vi "Alter Display.vi"(7 "obsticle location":dbl[](array[numeric]), 8 "error in (no error)":errorcluster, 9 "Display Map":dbl[][](array[numeric]), 10 "robot direction":string, 11 "robot location":dbl[](array[numeric])) -> (0 "error out":errorcluster, 2 "Map":u16[][](array[ring]), 3 "target location":dbl[](array[numeric]))   [LabVIEW 2015]
uses:
  <vilib>/robotics/Navigation/shared/WorldMap/OccupancyGridWorldMap/NI_Robotics_OccupancyGridWorldMap.lvclass
  <vilib>/robotics/Navigation/NI_Robotics_Navigation .lvlib
panel:
  out "Indices":i32[][](array[numeric])
  out "distances":dbl[](array[numeric])
  out "Priority level array":dbl[][](array[numeric])
  out "route map":dbl[][](array[numeric])
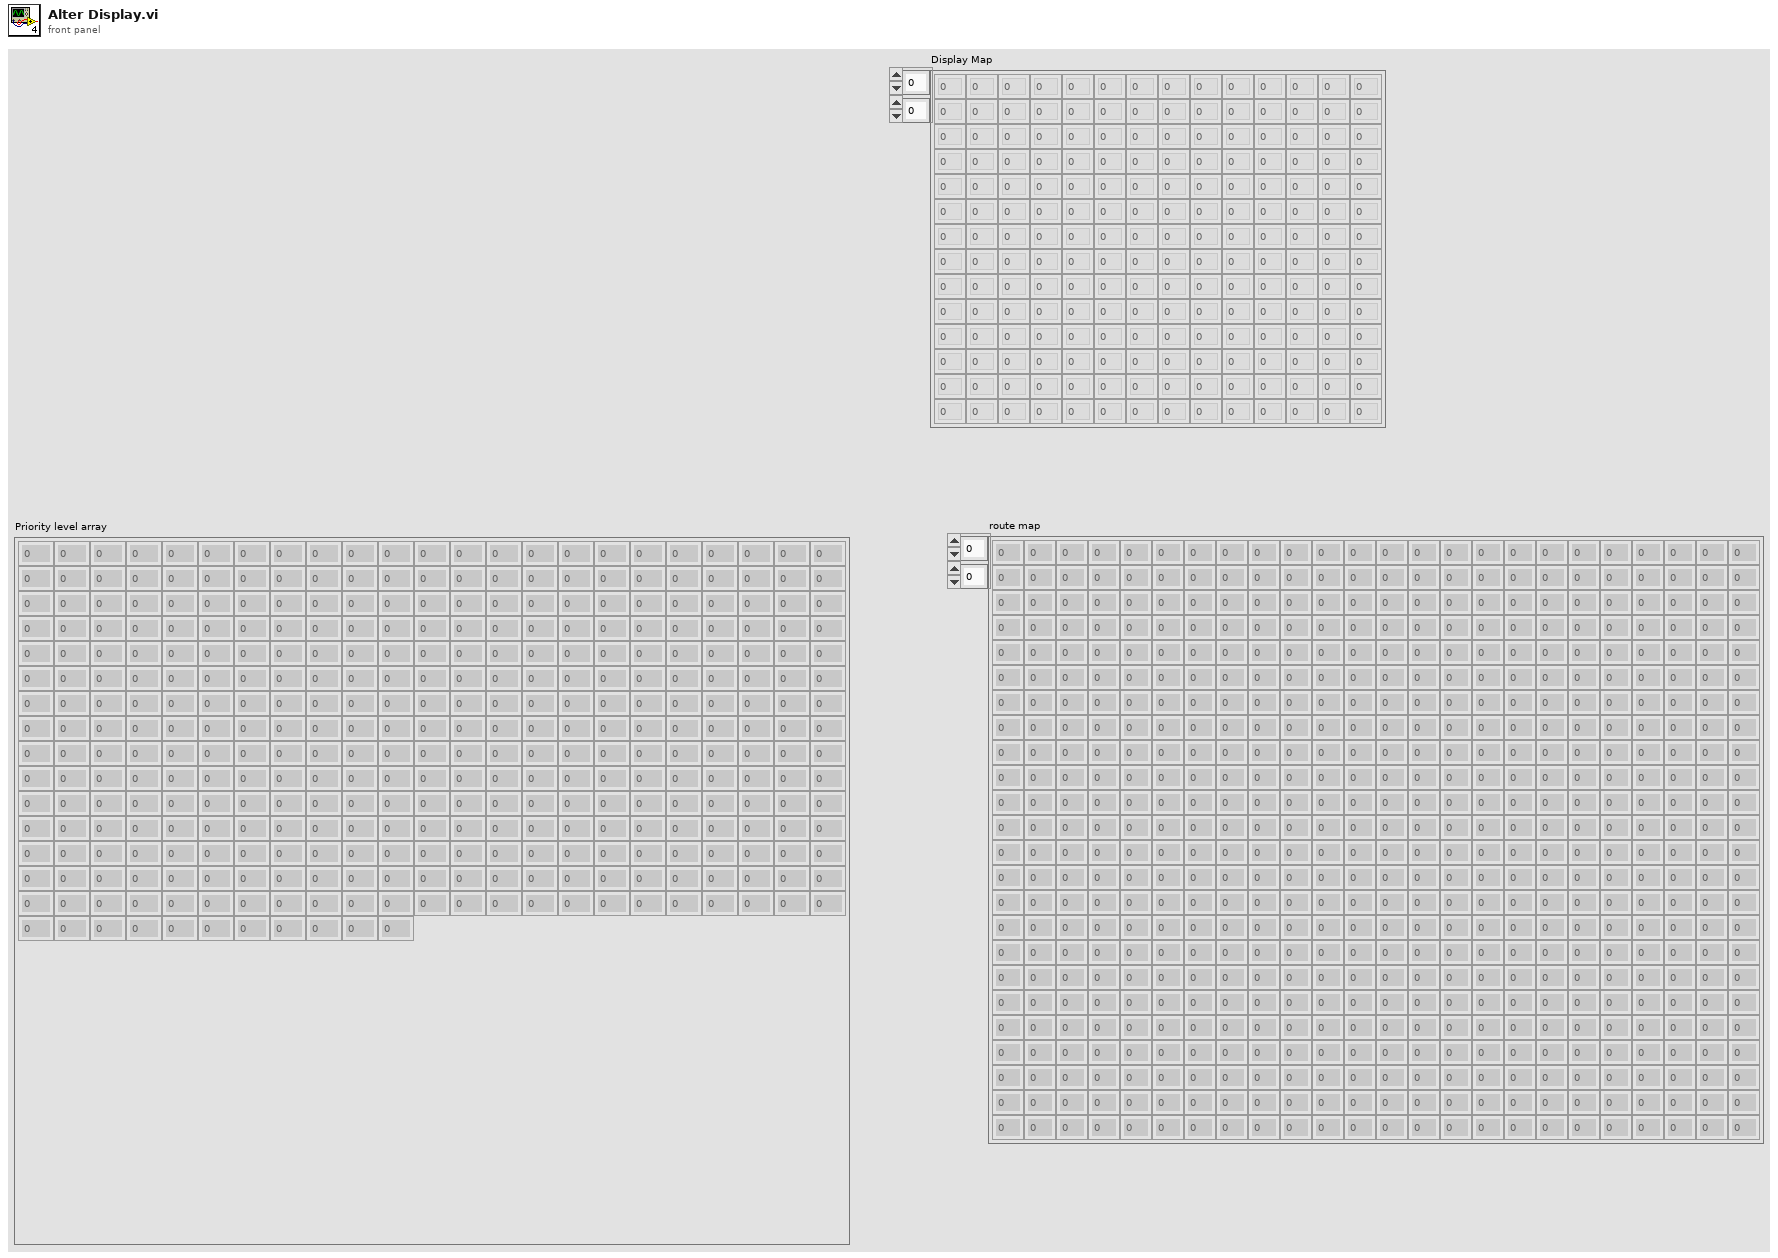
[diagram p1: front panel]
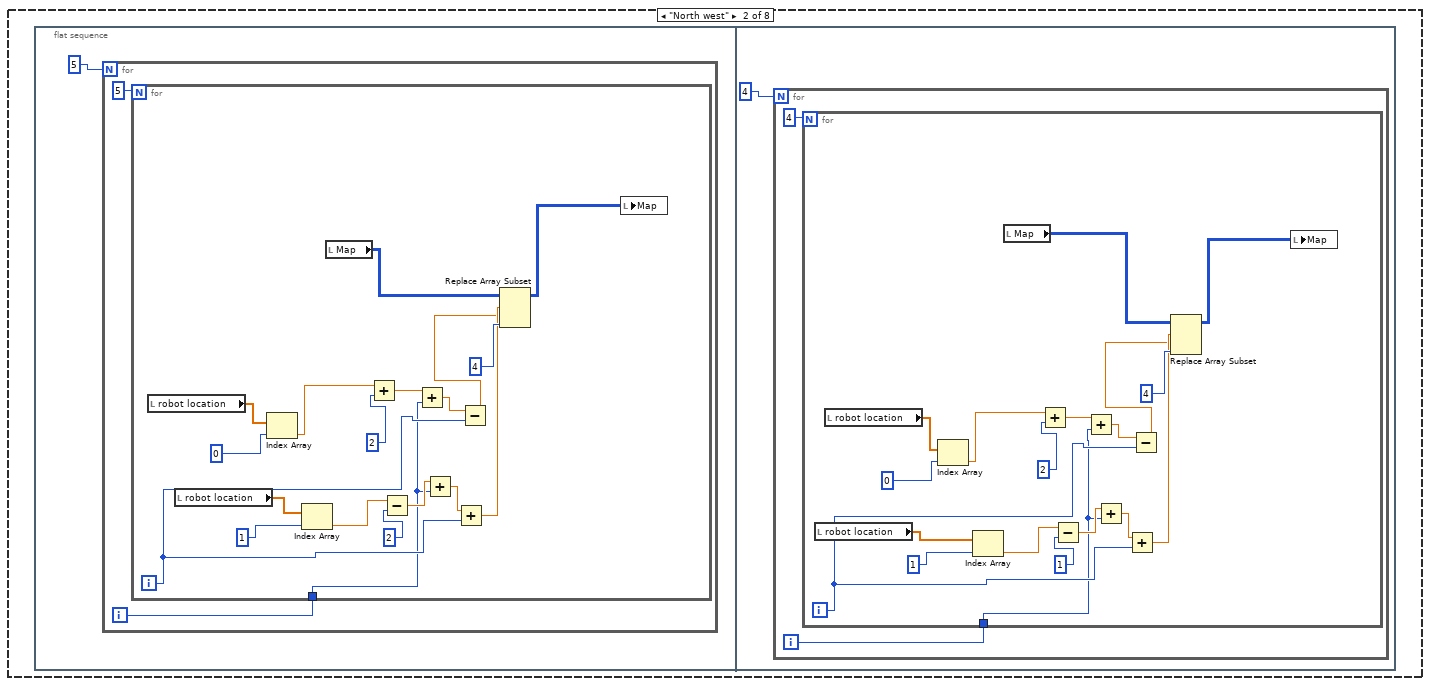
[diagram p2: hidden frame]
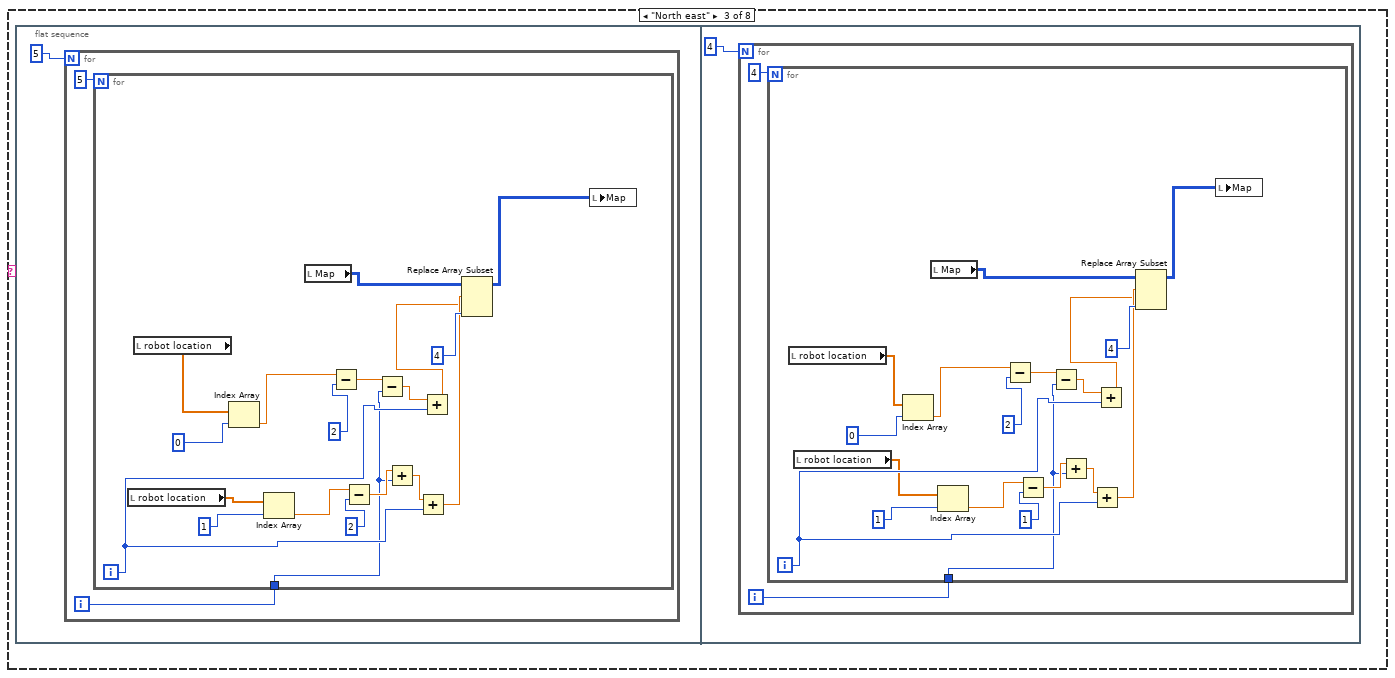
[diagram p3: hidden frame]
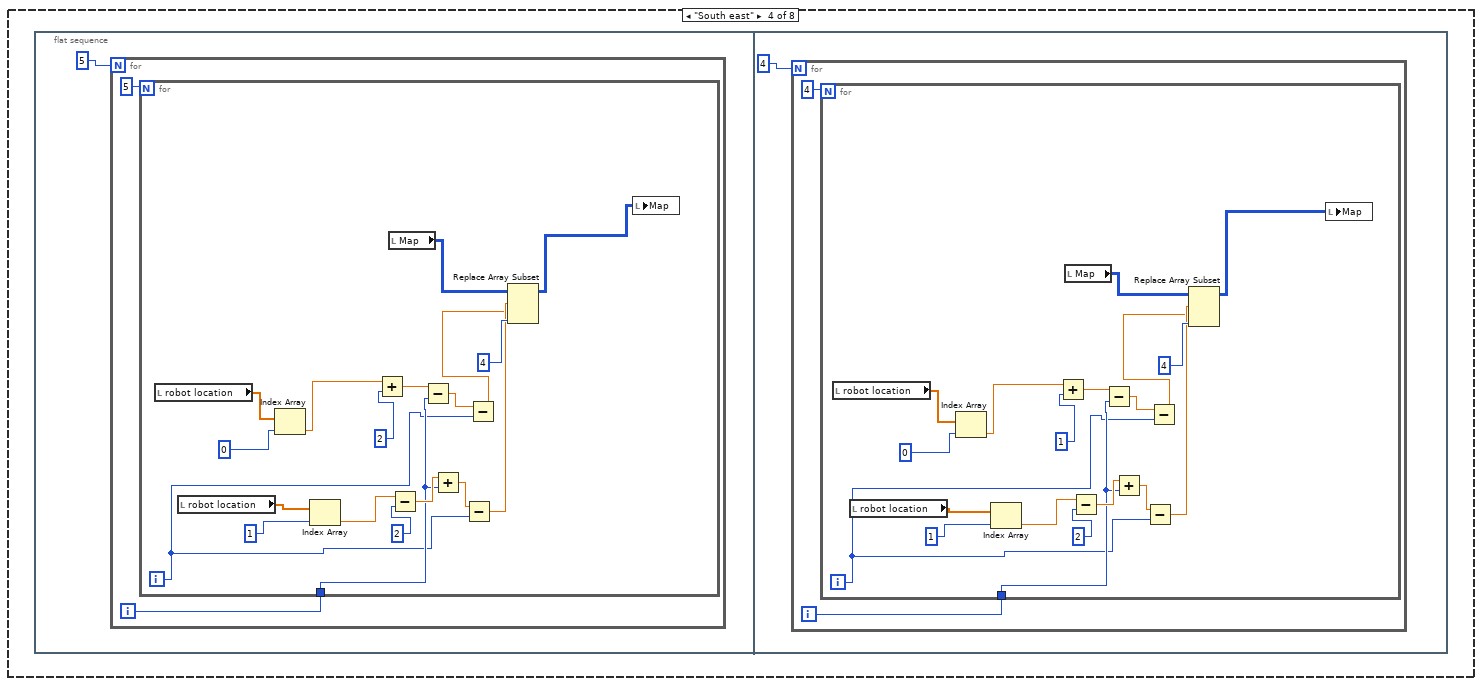
[diagram p4: hidden frame]
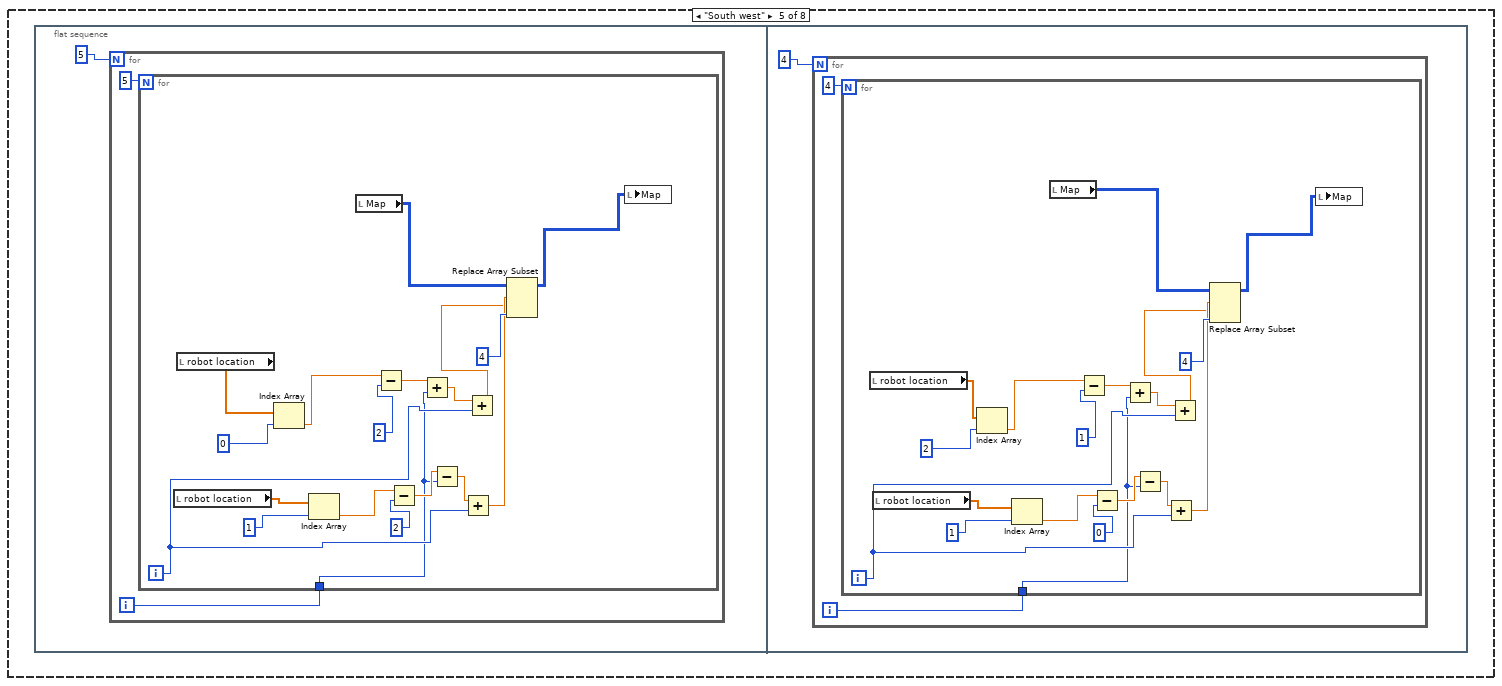
[diagram p5: hidden frame]
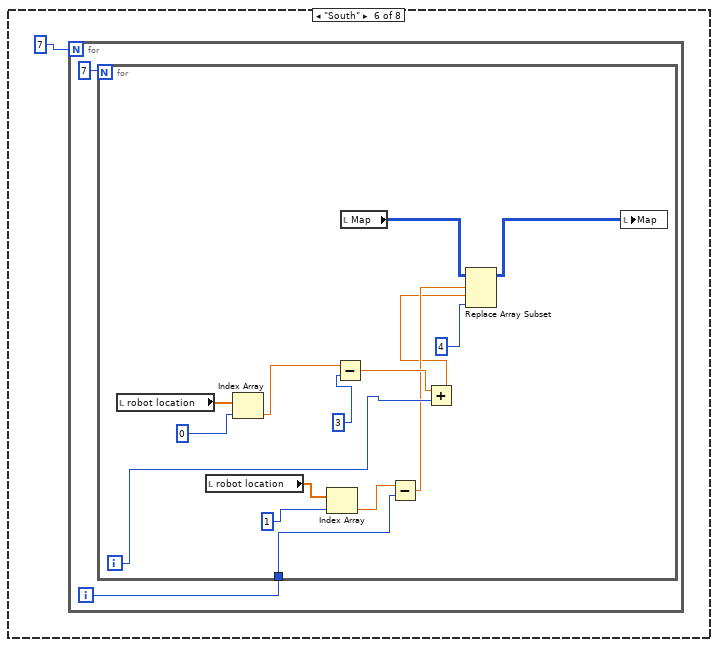
[diagram p6: hidden frame]
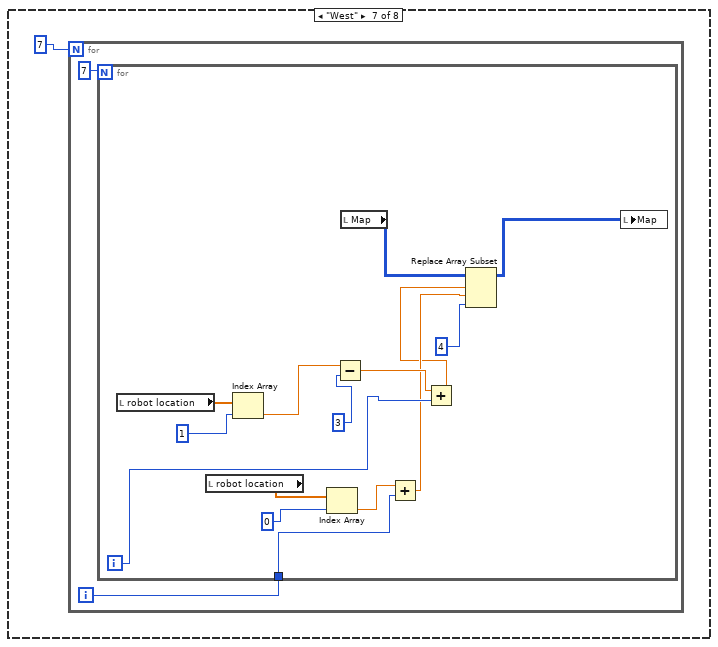
[diagram p7: hidden frame]
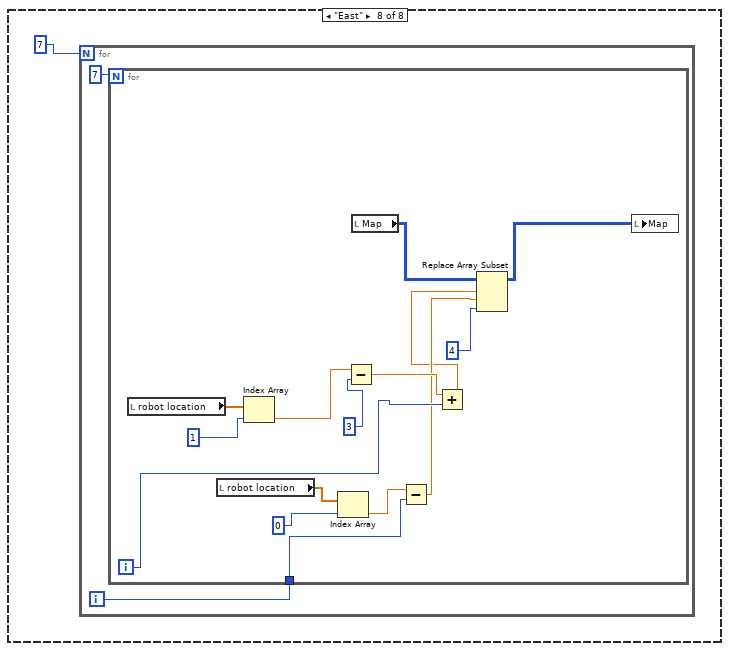
[diagram p8: hidden frame]
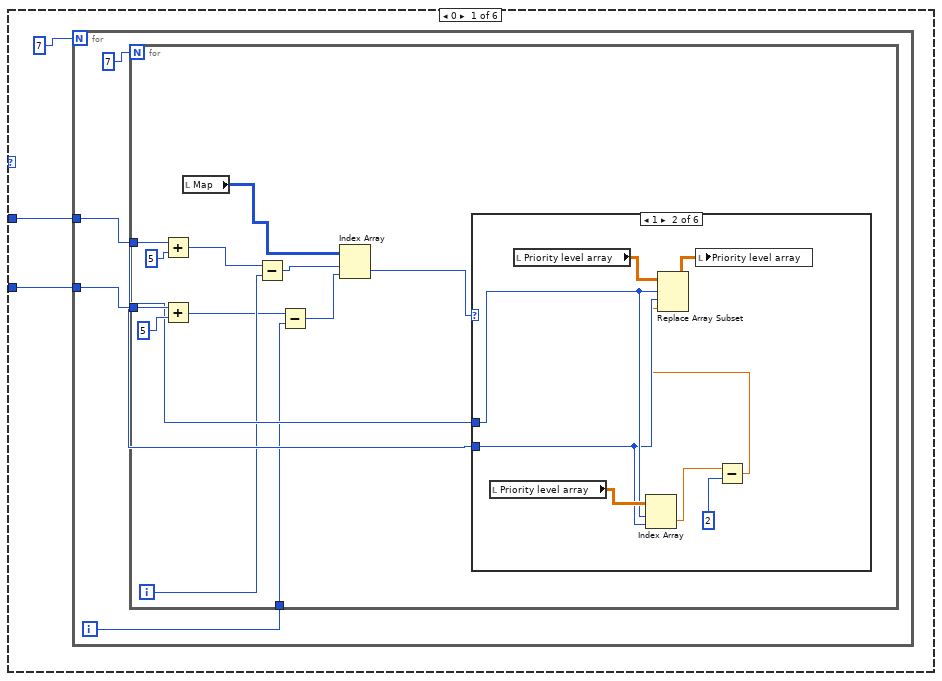
[diagram p9: hidden frame]
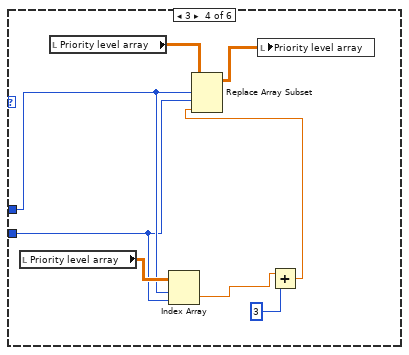
[diagram p12: hidden frame]
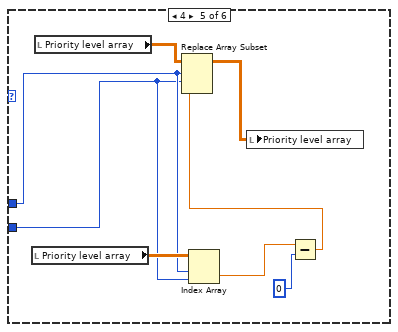
[diagram p13: hidden frame]
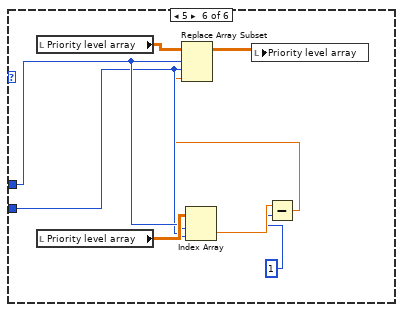
[diagram p14: hidden frame]
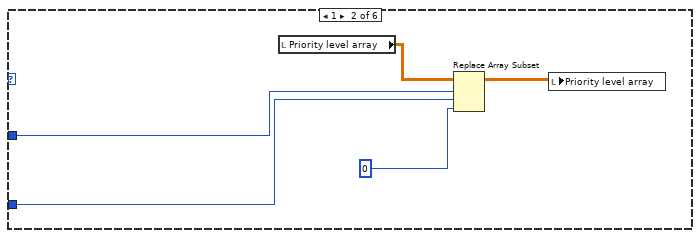
[diagram p15: hidden frame]
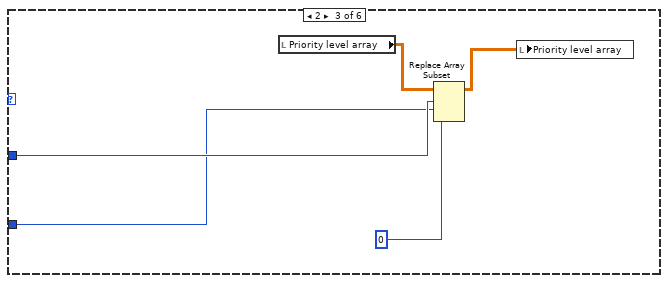
[diagram p16: hidden frame]
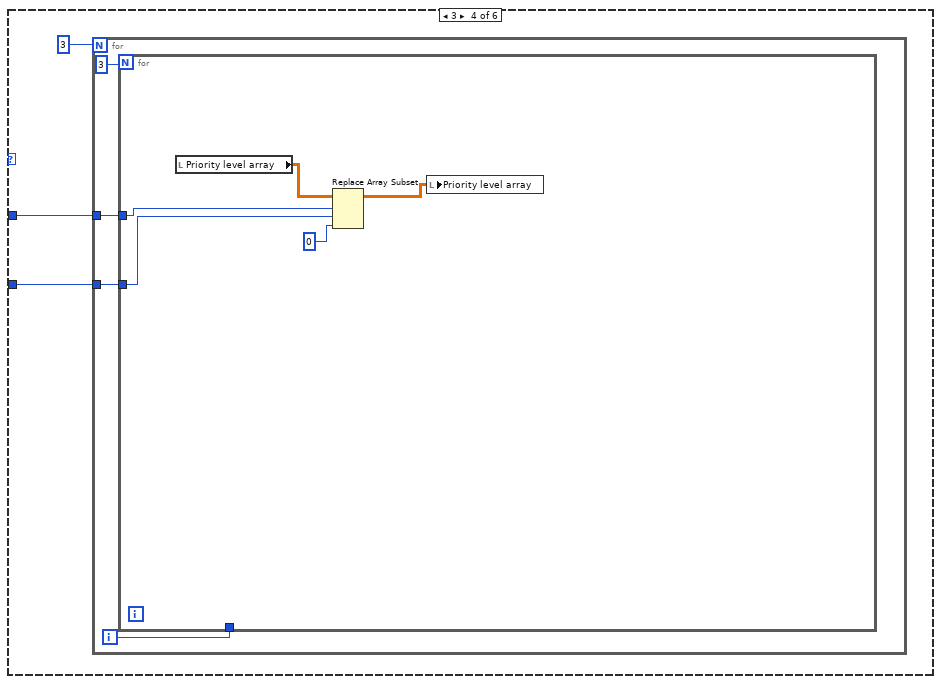
[diagram p17: hidden frame]
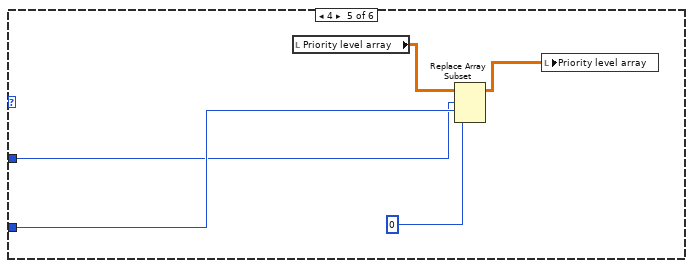
[diagram p18: hidden frame]
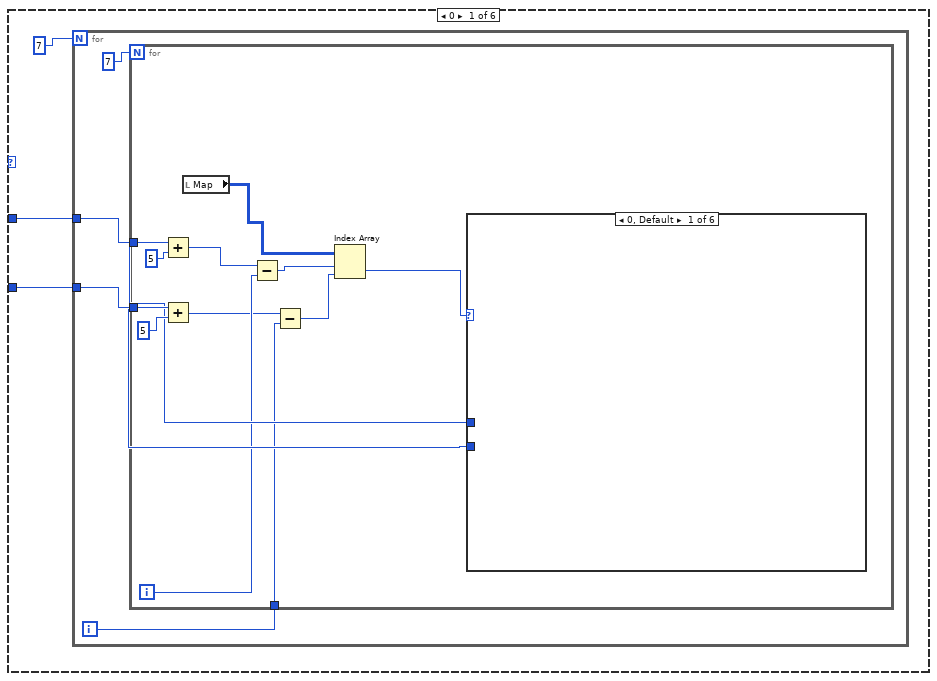
[diagram p20: hidden frame]
diagram:
  n1 = flat-sequence {
    tunnel: "error in (no error)" -> [w2]
    frame #0 {
      "Map" <- "Display Map"
      "Priority level array" <- "Display Map"
      "route map" <- "Display Map"
      "error out" <- w2
    }
    frame #1 {
      n2 = for {
        N: 40 -> [_]
        i -> [w5]
        n3 = for {
          N: 40 -> [_]
          tunnel: w5 -> [w11]
          i -> [w12]
          n4 = local read "Priority level array"() -> (w7:dbl[][])
          n5 = local read "route map"() -> (w8:dbl[][])
          n6 = Replace Array Subset(array=w8, new element=0, index (row)=w12, index (col)=w11) -> (w13:dbl[][])
          n7 = Replace Array Subset(array=w7, new element=15, index (row)=w12, index (col)=w11) -> (w14:dbl[][])
          n8 = local write "Priority level array"(w14) -> ()
          n9 = local write "route map"(w13) -> ()
        }
      }
    }
    frame #2 {
      n10 = case shown="\"North\", Default" "robot direction" {
        frame "North", Default {
          n11 = for {
            N: 7 -> [_]
            i -> [w17]
            n12 = for {
              N: 7 -> [_]
              tunnel: w17 -> [w25]
              i -> [w29]
              n13 = local read "robot location"() -> (w20:dbl[])
              n14 = local read "robot location"() -> (w19:dbl[])
              n15 = Index Array(array=w20, index=0) -> (element=w22:dbl)
              n16 = Index Array(array=w19, index=1) -> (element=w21:dbl)
              n17 = Subtract(x=w22, y=3) -> (x-y=w28:dbl)
              n18 = local read "Map"() -> (w24:u16[][])
              n19 = Add(x=w21, y=w25) -> (x+y=w27:dbl)
              n20 = Add(x=w28, y=w29) -> (x+y=w26:dbl)
              n21 = Replace Array Subset(array=w24, new element=4, index (row)=w27, index (col)=w26) -> (w23:u16[][])
              n22 = local write "Map"(w23) -> ()
            }
          }
        }
        frame "North west" {
          n23 = flat-sequence {
            frame #0 {
              n24 = for {
                N: 5 -> [_]
                i -> [w35]
                n25 = for {
                  N: 5 -> [_]
                  tunnel: w35 -> [w37]
                  i -> [w48]
                  n26 = local read "robot location"() -> (w43:dbl[])
                  n27 = local read "robot location"() -> (w42:dbl[])
                  n28 = Index Array(array=w43, index=0) -> (element=w49:dbl)
                  n29 = Index Array(array=w42, index=1) -> (element=w47:dbl)
                  n30 = local read "Map"() -> (w41:u16[][])
                  n31 = Add(x=w49, y=2) -> (x+y=w39:dbl)
                  n32 = Subtract(x=w47, y=2) -> (x-y=w45:dbl)
                  n33 = Add(x=w39, y=w37) -> (x+y=w38:dbl)
                  n34 = Add(x=w45, y=w37) -> (x+y=w44:dbl)
                  n35 = Add(x=w44, y=w48) -> (x+y=w51:dbl)
                  n36 = Subtract(x=w38, y=w48) -> (x-y=w50:dbl)
                  n37 = Replace Array Subset(array=w41, new element=4, index (row)=w51, index (col)=w50) -> (w40:u16[][])
                  n38 = local write "Map"(w40) -> ()
                }
              }
            }
            frame #1 {
              n39 = for {
                N: 4 -> [_]
                i -> [w57]
                n40 = for {
                  N: 4 -> [_]
                  tunnel: w57 -> [w64]
                  i -> [w70]
                  n41 = local read "robot location"() -> (w59:dbl[])
                  n42 = local read "robot location"() -> (w60:dbl[])
                  n43 = Index Array(array=w60, index=0) -> (element=w71:dbl)
                  n44 = Index Array(array=w59, index=1) -> (element=w69:dbl)
                  n45 = local read "Map"() -> (w62:u16[][])
                  n46 = Add(x=w71, y=2) -> (x+y=w67:dbl)
                  n47 = Subtract(x=w69, y=1) -> (x-y=w66:dbl)
                  n48 = Add(x=w67, y=w64) -> (x+y=w65:dbl)
                  n49 = Add(x=w66, y=w64) -> (x+y=w63:dbl)
                  n50 = Add(x=w63, y=w70) -> (x+y=w73:dbl)
                  n51 = Subtract(x=w65, y=w70) -> (x-y=w72:dbl)
                  n52 = Replace Array Subset(array=w62, new element=4, index (row)=w73, index (col)=w72) -> (w61:u16[][])
                  n53 = local write "Map"(w61) -> ()
                }
              }
            }
          }
        }
        frame "North east" {
          n54 = flat-sequence {
            frame #0 {
              n55 = for {
                N: 5 -> [_]
                i -> [w79]
                n56 = for {
                  N: 5 -> [_]
                  tunnel: w79 -> [w86]
                  i -> [w92]
                  n57 = local read "robot location"() -> (w81:dbl[])
                  n58 = local read "robot location"() -> (w82:dbl[])
                  n59 = Index Array(array=w82, index=0) -> (element=w93:dbl)
                  n60 = Index Array(array=w81, index=1) -> (element=w91:dbl)
                  n61 = local read "Map"() -> (w83:u16[][])
                  n62 = Subtract(x=w93, y=2) -> (x-y=w89:dbl)
                  n63 = Subtract(x=w91, y=2) -> (x-y=w88:dbl)
                  n64 = Subtract(x=w89, y=w86) -> (x-y=w87:dbl)
                  n65 = Add(x=w88, y=w86) -> (x+y=w85:dbl)
                  n66 = Add(x=w85, y=w92) -> (x+y=w95:dbl)
                  n67 = Add(x=w87, y=w92) -> (x+y=w94:dbl)
                  n68 = Replace Array Subset(array=w83, new element=4, index (row)=w95, index (col)=w94) -> (w84:u16[][])
                  n69 = local write "Map"(w84) -> ()
                }
              }
            }
            frame #1 {
              n70 = for {
                N: 4 -> [_]
                i -> [w101]
                n71 = for {
                  N: 4 -> [_]
                  tunnel: w101 -> [w103]
                  i -> [w114]
                  n72 = local read "robot location"() -> (w105:dbl[])
                  n73 = local read "robot location"() -> (w104:dbl[])
                  n74 = Index Array(array=w105, index=0) -> (element=w115:dbl)
                  n75 = local read "Map"() -> (w107:u16[][])
                  n76 = Index Array(array=w104, index=1) -> (element=w113:dbl)
                  n77 = Subtract(x=w115, y=2) -> (x-y=w111:dbl)
                  n78 = Subtract(x=w113, y=1) -> (x-y=w110:dbl)
                  n79 = Subtract(x=w111, y=w103) -> (x-y=w109:dbl)
                  n80 = Add(x=w110, y=w103) -> (x+y=w108:dbl)
                  n81 = Add(x=w108, y=w114) -> (x+y=w117:dbl)
                  n82 = Add(x=w109, y=w114) -> (x+y=w116:dbl)
                  n83 = Replace Array Subset(array=w107, new element=4, index (row)=w117, index (col)=w116) -> (w106:u16[][])
                  n84 = local write "Map"(w106) -> ()
                }
              }
            }
          }
        }
        frame "South east" {
          n85 = flat-sequence {
            frame #0 {
              n86 = for {
                N: 5 -> [_]
                i -> [w123]
                n87 = for {
                  N: 5 -> [_]
                  tunnel: w123 -> [w131]
                  i -> [w125]
                  n88 = local read "robot location"() -> (w127:dbl[])
                  n89 = local read "robot location"() -> (w126:dbl[])
                  n90 = Index Array(array=w127, index=0) -> (element=w137:dbl)
                  n91 = Index Array(array=w126, index=1) -> (element=w136:dbl)
                  n92 = Add(x=w137, y=2) -> (x+y=w134:dbl)
                  n93 = local read "Map"() -> (w128:u16[][])
                  n94 = Subtract(x=w136, y=2) -> (x-y=w133:dbl)
                  n95 = Subtract(x=w134, y=w131) -> (x-y=w132:dbl)
                  n96 = Add(x=w133, y=w131) -> (x+y=w130:dbl)
                  n97 = Subtract(x=w130, y=w125) -> (x-y=w139:dbl)
                  n98 = Subtract(x=w132, y=w125) -> (x-y=w138:dbl)
                  n99 = Replace Array Subset(array=w128, new element=4, index (row)=w139, index (col)=w138) -> (w129:u16[][])
                  n100 = local write "Map"(w129) -> ()
                }
              }
            }
            frame #1 {
              n101 = for {
                N: 4 -> [_]
                i -> [w145]
                n102 = for {
                  N: 4 -> [_]
                  tunnel: w145 -> [w153]
                  i -> [w150]
                  n103 = local read "robot location"() -> (w151:dbl[])
                  n104 = local read "robot location"() -> (w149:dbl[])
                  n105 = Index Array(array=w151, index=0) -> (element=w159:dbl)
                  n106 = Index Array(array=w149, index=1) -> (element=w158:dbl)
                  n107 = Add(x=w159, y=1) -> (x+y=w156:dbl)
                  n108 = local read "Map"() -> (w148:u16[][])
                  n109 = Subtract(x=w158, y=2) -> (x-y=w155:dbl)
                  n110 = Subtract(x=w156, y=w153) -> (x-y=w154:dbl)
                  n111 = Add(x=w155, y=w153) -> (x+y=w152:dbl)
                  n112 = Subtract(x=w152, y=w150) -> (x-y=w161:dbl)
                  n113 = Subtract(x=w154, y=w150) -> (x-y=w160:dbl)
                  n114 = Replace Array Subset(array=w148, new element=4, index (row)=w161, index (col)=w160) -> (w147:u16[][])
                  n115 = local write "Map"(w147) -> ()
                }
              }
            }
          }
        }
        frame "South west" {
          n116 = flat-sequence {
            frame #0 {
              n117 = for {
                N: 5 -> [_]
                i -> [w167]
                n118 = for {
                  N: 5 -> [_]
                  tunnel: w167 -> [w175]
                  i -> [w181]
                  n119 = local read "robot location"() -> (w170:dbl[])
                  n120 = local read "robot location"() -> (w171:dbl[])
                  n121 = Index Array(array=w171, index=0) -> (element=w169:dbl)
                  n122 = Index Array(array=w170, index=1) -> (element=w180:dbl)
                  n123 = local read "Map"() -> (w172:u16[][])
                  n124 = Subtract(x=w169, y=2) -> (x-y=w178:dbl)
                  n125 = Subtract(x=w180, y=2) -> (x-y=w177:dbl)
                  n126 = Add(x=w178, y=w175) -> (x+y=w176:dbl)
                  n127 = Subtract(x=w177, y=w175) -> (x-y=w174:dbl)
                  n128 = Add(x=w174, y=w181) -> (x+y=w183:dbl)
                  n129 = Add(x=w176, y=w181) -> (x+y=w182:dbl)
                  n130 = Replace Array Subset(array=w172, new element=4, index (row)=w183, index (col)=w182) -> (w173:u16[][])
                  n131 = local write "Map"(w173) -> ()
                }
              }
            }
            frame #1 {
              n132 = for {
                N: 4 -> [_]
                i -> [w189]
                n133 = for {
                  N: 4 -> [_]
                  tunnel: w189 -> [w196]
                  i -> [w202]
                  n134 = local read "robot location"() -> (w192:dbl[])
                  n135 = local read "robot location"() -> (w191:dbl[])
                  n136 = Index Array(array=w192, index=2) -> (element=w203:dbl)
                  n137 = Index Array(array=w191, index=1) -> (element=w201:dbl)
                  n138 = local read "Map"() -> (w194:u16[][])
                  n139 = Subtract(x=w203, y=1) -> (x-y=w199:dbl)
                  n140 = Subtract(x=w201, y=0) -> (x-y=w198:dbl)
                  n141 = Add(x=w199, y=w196) -> (x+y=w197:dbl)
                  n142 = Subtract(x=w198, y=w196) -> (x-y=w195:dbl)
                  n143 = Add(x=w195, y=w202) -> (x+y=w205:dbl)
                  n144 = Add(x=w197, y=w202) -> (x+y=w204:dbl)
                  n145 = Replace Array Subset(array=w194, new element=4, index (row)=w205, index (col)=w204) -> (w193:u16[][])
                  n146 = local write "Map"(w193) -> ()
                }
              }
            }
          }
        }
        frame "South" {
          n147 = for {
            N: 7 -> [_]
            i -> [w211]
            n148 = for {
              N: 7 -> [_]
              tunnel: w211 -> [w219]
              i -> [w223]
              n149 = local read "robot location"() -> (w216:dbl[])
              n150 = local read "robot location"() -> (w215:dbl[])
              n151 = Index Array(array=w216, index=0) -> (element=w214:dbl)
              n152 = Index Array(array=w215, index=1) -> (element=w213:dbl)
              n153 = Subtract(x=w214, y=3) -> (x-y=w222:dbl)
              n154 = local read "Map"() -> (w218:u16[][])
              n155 = Subtract(x=w213, y=w219) -> (x-y=w221:dbl)
              n156 = Add(x=w222, y=w223) -> (x+y=w220:dbl)
              n157 = Replace Array Subset(array=w218, new element=4, index (row)=w221, index (col)=w220) -> (w217:u16[][])
              n158 = local write "Map"(w217) -> ()
            }
          }
        }
        frame "West" {
          n159 = for {
            N: 7 -> [_]
            i -> [w229]
            n160 = for {
              N: 7 -> [_]
              tunnel: w229 -> [w239]
              i -> [w241]
              n161 = local read "robot location"() -> (w234:dbl[])
              n162 = local read "robot location"() -> (w233:dbl[])
              n163 = Index Array(array=w234, index=1) -> (element=w232:dbl)
              n164 = Index Array(array=w233, index=0) -> (element=w231:dbl)
              n165 = Subtract(x=w232, y=3) -> (x-y=w240:dbl)
              n166 = local read "Map"() -> (w236:u16[][])
              n167 = Add(x=w231, y=w239) -> (x+y=w238:dbl)
              n168 = Add(x=w240, y=w241) -> (x+y=w237:dbl)
              n169 = Replace Array Subset(array=w236, new element=4, index (row)=w237, index (col)=w238) -> (w235:u16[][])
              n170 = local write "Map"(w235) -> ()
            }
          }
        }
        frame "East" {
          n171 = for {
            N: 7 -> [_]
            i -> [w247]
            n172 = for {
              N: 7 -> [_]
              tunnel: w247 -> [w251]
              i -> [w253]
              n173 = local read "robot location"() -> (w260:dbl[])
              n174 = local read "robot location"() -> (w258:dbl[])
              n175 = Index Array(array=w260, index=1) -> (element=w255:dbl)
              n176 = Index Array(array=w258, index=0) -> (element=w256:dbl)
              n177 = Subtract(x=w255, y=3) -> (x-y=w252:dbl)
              n178 = local read "Map"() -> (w263:u16[][])
              n179 = Subtract(x=w256, y=w251) -> (x-y=w250:dbl)
              n180 = Add(x=w252, y=w253) -> (x+y=w249:dbl)
              n181 = Replace Array Subset(array=w263, new element=4, index (row)=w249, index (col)=w250) -> (w262:u16[][])
              n182 = local write "Map"(w262) -> ()
            }
          }
        }
      }
    }
    frame #3 {
      n183 = Index Array(array="obsticle location", index #1=0, index #2=1) -> (element #1=w266:dbl, element #2=w265:dbl)
      n184 = for {
        N: 3 -> [_]
        tunnel: w266 -> [w271]
        tunnel: w265 -> [w270]
        i -> [w273]
        n185 = for {
          N: 3 -> [_]
          tunnel: w273 -> [w276]
          tunnel: w271 -> [w275]
          tunnel: w270 -> [w274]
          i -> [w280]
          n186 = Subtract(x=w274, y=1) -> (x-y=w282:dbl)
          n187 = Add(x=w282, y=w280) -> (x+y=w281:dbl)
          n188 = Subtract(x=w275, y=1) -> (x-y=w279:dbl)
          n189 = local read "Map"() -> (w286:u16[][])
          n190 = Add(x=w279, y=w276) -> (x+y=w278:dbl)
          n191 = Replace Array Subset(array=w286, new element=1, index (row)=w281, index (col)=w278) -> (w285:u16[][])
          n192 = local write "Map"(w285) -> ()
        }
      }
    }
    frame #4 {
      n193 = for {
        N: 40 -> [_]
        i -> [w288]
        n194 = for {
          N: 40 -> [_]
          tunnel: w288 -> [w292]
          i -> [w291]
          n195 = local read "Map"() -> (w293:u16[][])
          n196 = Index Array(array=w293, index (row)=w291, index (col)=w292) -> (element=w290:u16)
          n197 = case shown="5, Default" w290 {
            tunnel: w292 -> [w296 w346 w352 w357 w369 w373]
            tunnel: w291 -> [w295 w345 w353 w356 w368 w374]
            frame 0 {
              n198 = for {
                N: 7 -> [_]
                tunnel: w296 -> [w300]
                tunnel: w295 -> [w299]
                i -> [w297]
                n199 = for {
                  N: 7 -> [_]
                  tunnel: w300 -> [w309]
                  tunnel: w299 -> [w308]
                  tunnel: w297 -> [w304]
                  i -> [w306]
                  n200 = Add(x=w308, y=5) -> (x+y=w307:i32)
                  n201 = Add(x=w309, y=5) -> (x+y=w305:i32)
                  n202 = local read "Map"() -> (w312:u16[][])
                  n203 = Subtract(x=w307, y=w306) -> (x-y=w302:i32)
                  n204 = Subtract(x=w305, y=w304) -> (x-y=w303:i32)
                  n205 = Index Array(array=w312, index (row)=w302, index (col)=w303) -> (element=w301:u16)
                  n206 = case shown="1" w301 {
                    tunnel: w309 -> [_ w316 _ w325 w332 w340]
                    tunnel: w308 -> [_ w317 _ w326 w333 w341]
                    frame 0, Default {
                    }
                    frame 1 {
                      n207 = local read "Priority level array"() -> (w320:dbl[][])
                      n208 = local read "Priority level array"() -> (w319:dbl[][])
                      n209 = Index Array(array=w320, index (row)=w317, index (col)=w316) -> (element=w315:dbl)
                      n210 = Subtract(x=w315, y=2) -> (x-y=w313:dbl)
                      n211 = Replace Array Subset(array=w319, new element=w313, index (row)=w317, index (col)=w316) -> (w318:dbl[][])
                      n212 = local write "Priority level array"(w318) -> ()
                    }
                    frame 2 {
                    }
                    frame 3 {
                      n213 = local read "Priority level array"() -> (w327:dbl[][])
                      n214 = local read "Priority level array"() -> (w328:dbl[][])
                      n215 = Index Array(array=w327, index (row)=w326, index (col)=w325) -> (element=w324:dbl)
                      n216 = Add(x=w324, y=3) -> (x+y=w322:dbl)
                      n217 = Replace Array Subset(array=w328, new element=w322, index (row)=w326, index (col)=w325) -> (w323:dbl[][])
                      n218 = local write "Priority level array"(w323) -> ()
                    }
                    frame 4 {
                      n219 = local read "Priority level array"() -> (w334:dbl[][])
                      n220 = local read "Priority level array"() -> (w336:dbl[][])
                      n221 = Index Array(array=w334, index (row)=w333, index (col)=w332) -> (element=w331:dbl)
                      n222 = Subtract(x=w331, y=0) -> (x-y=w330:dbl)
                      n223 = Replace Array Subset(array=w336, new element=w330, index (row)=w333, index (col)=w332) -> (w335:dbl[][])
                      n224 = local write "Priority level array"(w335) -> ()
                    }
                    frame 5 {
                      n225 = local read "Priority level array"() -> (w342:dbl[][])
                      n226 = local read "Priority level array"() -> (w344:dbl[][])
                      n227 = Index Array(array=w344, index (row)=w341, index (col)=w340) -> (element=w339:dbl)
                      n228 = Subtract(x=w339, y=1) -> (x-y=w338:dbl)
                      n229 = Replace Array Subset(array=w342, new element=w338, index (row)=w341, index (col)=w340) -> (w343:dbl[][])
                      n230 = local write "Priority level array"(w343) -> ()
                    }
                  }
                }
              }
            }
            frame 1 {
              n231 = local read "Priority level array"() -> (w349:dbl[][])
              n232 = Replace Array Subset(array=w349, new element=0, index (row)=w345, index (col)=w346) -> (w348:dbl[][])
              n233 = local write "Priority level array"(w348) -> ()
            }
            frame 2 {
              n234 = local read "Priority level array"() -> (w354:dbl[][])
              n235 = Replace Array Subset(array=w354, new element=0, index (row)=w353, index (col)=w352) -> (w351:dbl[][])
              n236 = local write "Priority level array"(w351) -> ()
            }
            frame 3 {
              n237 = for {
                N: 3 -> [_]
                tunnel: w357 -> [w361]
                tunnel: w356 -> [w360]
                i -> [w358]
                n238 = for {
                  N: 3 -> [_]
                  tunnel: w361 -> [w362]
                  tunnel: w360 -> [w363]
                  tunnel: w358 -> [_]
                  n239 = local read "Priority level array"() -> (w366:dbl[][])
                  n240 = Replace Array Subset(array=w366, new element=0, index (row)=w363, index (col)=w362) -> (w365:dbl[][])
                  n241 = local write "Priority level array"(w365) -> ()
                }
              }
            }
            frame 4 {
              n242 = local read "Priority level array"() -> (w371:dbl[][])
              n243 = Replace Array Subset(array=w371, new element=0, index (row)=w368, index (col)=w369) -> (w370:dbl[][])
              n244 = local write "Priority level array"(w370) -> ()
            }
            frame 5, Default {
              n245 = local read "Priority level array"() -> (w376:dbl[][])
              n246 = Replace Array Subset(array=w376, new element=0, index (row)=w374, index (col)=w373) -> (w375:dbl[][])
              n247 = local write "Priority level array"(w375) -> ()
            }
          }
        }
      }
    }
    frame #5 {
      n248 = local read "Priority level array"() -> (w378:dbl[][])
      n249 = for {
        tunnel: [w381] -> _ mode=indexing
        shift-right: [w385] -> w380
        shift-left: i32[][] [] -> [w383]
        tunnel: w378 -> [w381] mode=indexing
        i -> [w387]
        n250 = Increment(x=w387) -> (x+1=w386:i32)
        n251 = for {
          tunnel: w381 -> [w396] mode=indexing
          tunnel: w386 -> [w392]
          shift-right: [w391] -> w384
          shift-left: i32[][] [] -> [w390]
          i -> [w394]
          n252 = local read "Priority level array"() -> (w389:dbl[][])
          n253 = Array Max & Min(array=w389) -> (max value=w388:dbl)  [unwired: 3 out]
          n254 = Equal?(x=w396, y=w388) -> (x = y?=w395:bool)
          n255 = Increment(x=w394) -> (x+1=w393:i32)
          n256 = case shown="True" w395 {
            tunnel: w393 -> [_ w402]
            tunnel: w392 -> [_ w401]
            tunnel: [w397 w399] -> w391
            tunnel: w390 -> [w397 w398]
            frame False {
            }
            frame True {
              n257 = Build Array(w402, w401) -> (w400:i32[])
              n258 = Build Array (concatenate)(w398, w400) -> (w399:i32[][])
            }
          }
        }
        n259 = Build Array (concatenate)(w383, w384) -> (w385:i32[][])
      }
      "Indices" <- w380
      "distances" <- i32[] [0, 0, 0, 0, 0, 0, 0, 0, 0, 0]
    }
    frame #6 {
      n260 = for {
        N: 10 -> [_]
        i -> [w406]
        n261 = local read "Indices"() -> (w427:i32[][])
        n262 = Index Array(array=w427, index (row)=w406, index (col)=0) -> (element=w420:i32)
        n263 = Index Array(array=w427, index (row)=w406, index (col)=1) -> (element=w419:i32)
        n264 = Index Array(array="robot location", index=1) -> (element=w422:dbl)
        n265 = Index Array(array="robot location", index=0) -> (element=w424:dbl)
        n266 = Add(x=w422, y=1) -> (x+y=w417:dbl)
        n267 = Add(x=w424, y=1) -> (x+y=w418:dbl)
        n268 = Subtract(x=w420, y=w418) -> (x-y=w416:dbl)
        n269 = Subtract(x=w419, y=w417) -> (x-y=w409:dbl)
        n270 = Square(x=w409) -> (x^2=w415:dbl)
        n271 = Square(x=w416) -> (x^2=w414:dbl)
        n272 = Add(x=w414, y=w415) -> (x+y=w413:dbl)
        n273 = local read "distances"() -> (w412:dbl[])
        n274 = Square Root(x=w413) -> (sqrt(x)=w410:dbl)
        n275 = Replace Array Subset(array=w412, new element=w410, index=w406) -> (w411:dbl[])
        n276 = local write "distances"(w411) -> ()
      }
      "target location" <- i32[] [0, 0]
    }
    frame #7 {
      n277 = local read "distances"() -> (w435:dbl[])
      n278 = local read "Indices"() -> (w428:i32[][])
      n279 = Array Max & Min(array=w435) -> (min index (indices)=w430:i32)  [unwired: 3 out]
      n280 = local read "target location"() -> (w432:dbl[])
      n281 = Index Array(array=w428, index (row)=w430, index (col)=0) -> (element=w433:i32)
      n282 = Replace Array Subset(array=w432, new element=w433, index=0) -> (w434:dbl[])
      n283 = local write "target location"(w434) -> ()
    }
    frame #8 {
      n284 = local read "distances"() -> (w442:dbl[])
      n285 = local read "Indices"() -> (w441:i32[][])
      n286 = Array Max & Min(array=w442) -> (min index (indices)=w443:i32)  [unwired: 3 out]
      n287 = local read "target location"() -> (w438:dbl[])
      n288 = Index Array(array=w441, index (row)=w443, index (col)=1) -> (element=w437:i32)
      n289 = Replace Array Subset(array=w438, new element=w437, index=1) -> (w436:dbl[])
      n290 = local write "target location"(w436) -> ()
    }
    frame #9 {
      n291 = local read "target location"() -> (w450:dbl[])
      n292 = Index Array(array=w450, index #1=0, index #2=1) -> (element #1=w447:dbl, element #2=w446:dbl)
      n293 = local read "Map"() -> (w453:u16[][])
      n294 = Decrement(x=w446) -> (x-1=w445:dbl)
      n295 = Decrement(x=w447) -> (x-1=w444:dbl)
      n296 = Replace Array Subset(array=w453, new element=4, index (row)=w445, index (col)=w444) -> (w452:u16[][])
      n297 = local write "Map"(w452) -> ()
    }
    frame #10 {
      n298 = for {
        N: 40 -> [_]
        i -> [w455]
        n299 = for {
          N: 40 -> [_]
          tunnel: w455 -> [w459]
          i -> [w458]
          n300 = local read "Map"() -> (w460:u16[][])
          n301 = Index Array(array=w460, index (row)=w458, index (col)=w459) -> (element=w457:u16)
          n302 = case shown="2" w457 {
            tunnel: w459 -> [w463 w513 w519 w524 w536 w540]
            tunnel: w458 -> [w462 w512 w520 w523 w535 w541]
            frame 0 {
              n303 = for {
                N: 7 -> [_]
                tunnel: w463 -> [w467]
                tunnel: w462 -> [w466]
                i -> [w464]
                n304 = for {
                  N: 7 -> [_]
                  tunnel: w467 -> [w476]
                  tunnel: w466 -> [w475]
                  tunnel: w464 -> [w471]
                  i -> [w473]
                  n305 = Add(x=w475, y=5) -> (x+y=w474:i32)
                  n306 = Add(x=w476, y=5) -> (x+y=w472:i32)
                  n307 = local read "Map"() -> (w479:u16[][])
                  n308 = Subtract(x=w474, y=w473) -> (x-y=w469:i32)
                  n309 = Subtract(x=w472, y=w471) -> (x-y=w470:i32)
                  n310 = Index Array(array=w479, index (row)=w469, index (col)=w470) -> (element=w468:u16)
                  n311 = case shown="0, Default" w468 {
                    tunnel: w476 -> [_ w483 _ w492 w499 w507]
                    tunnel: w475 -> [_ w484 _ w493 w500 w508]
                    frame 0, Default {
                    }
                    frame 1 {
                      n312 = local read "route map"() -> (w487:dbl[][])
                      n313 = local read "route map"() -> (w486:dbl[][])
                      n314 = Index Array(array=w487, index (row)=w484, index (col)=w483) -> (element=w482:dbl)
                      n315 = Add(x=w482, y=2) -> (x+y=w480:dbl)
                      n316 = Replace Array Subset(array=w486, new element=w480, index (row)=w484, index (col)=w483) -> (w485:dbl[][])
                      n317 = local write "route map"(w485) -> ()
                    }
                    frame 2 {
                    }
                    frame 3 {
                      n318 = local read "route map"() -> (w494:dbl[][])
                      n319 = local read "route map"() -> (w495:dbl[][])
                      n320 = Index Array(array=w494, index (row)=w493, index (col)=w492) -> (element=w491:dbl)
                      n321 = Add(x=w491, y=0) -> (x+y=w489:dbl)
                      n322 = Replace Array Subset(array=w495, new element=w489, index (row)=w493, index (col)=w492) -> (w490:dbl[][])
                      n323 = local write "route map"(w490) -> ()
                    }
                    frame 4 {
                      n324 = local read "route map"() -> (w501:dbl[][])
                      n325 = local read "route map"() -> (w503:dbl[][])
                      n326 = Index Array(array=w501, index (row)=w500, index (col)=w499) -> (element=w498:dbl)
                      n327 = Add(x=w498, y=1) -> (x+y=w497:dbl)
                      n328 = Replace Array Subset(array=w503, new element=w497, index (row)=w500, index (col)=w499) -> (w502:dbl[][])
                      n329 = local write "route map"(w502) -> ()
                    }
                    frame 5 {
                      n330 = local read "route map"() -> (w509:dbl[][])
                      n331 = local read "route map"() -> (w511:dbl[][])
                      n332 = Index Array(array=w511, index (row)=w508, index (col)=w507) -> (element=w506:dbl)
                      n333 = Add(x=w506, y=1) -> (x+y=w505:dbl)
                      n334 = Replace Array Subset(array=w509, new element=w505, index (row)=w508, index (col)=w507) -> (w510:dbl[][])
                      n335 = local write "route map"(w510) -> ()
                    }
                  }
                }
              }
            }
            frame 1 {
              n336 = local read "route map"() -> (w516:dbl[][])
              n337 = Replace Array Subset(array=w516, new element=100, index (row)=w512, index (col)=w513) -> (w515:dbl[][])
              n338 = local write "route map"(w515) -> ()
            }
            frame 2 {
              n339 = local read "route map"() -> (w521:dbl[][])
              n340 = Replace Array Subset(array=w521, new element=0, index (row)=w520, index (col)=w519) -> (w518:dbl[][])
              n341 = local write "route map"(w518) -> ()
            }
            frame 3 {
              n342 = for {
                N: 3 -> [_]
                tunnel: w524 -> [w528]
                tunnel: w523 -> [w527]
                i -> [w525]
                n343 = for {
                  N: 3 -> [_]
                  tunnel: w528 -> [w529]
                  tunnel: w527 -> [w530]
                  tunnel: w525 -> [_]
                  n344 = local read "route map"() -> (w533:dbl[][])
                  n345 = Replace Array Subset(array=w533, new element=25, index (row)=w530, index (col)=w529) -> (w532:dbl[][])
                  n346 = local write "route map"(w532) -> ()
                }
              }
            }
            frame 4 {
              n347 = local read "route map"() -> (w538:dbl[][])
              n348 = Replace Array Subset(array=w538, new element=50, index (row)=w535, index (col)=w536) -> (w537:dbl[][])
              n349 = local write "route map"(w537) -> ()
            }
            frame 5, Default {
              n350 = local read "route map"() -> (w543:dbl[][])
              n351 = Replace Array Subset(array=w543, new element=50, index (row)=w541, index (col)=w540) -> (w542:dbl[][])
              n352 = local write "route map"(w542) -> ()
            }
          }
        }
      }
    }
    frame #11 {
      n353 = local read "route map"() -> (w556:dbl[][])
      n354 = local read "robot location"() -> (w555:dbl[])
      n355 = Multiply(x=w556, y=99) -> (x*y=w567:dbl[][])
      n356 = Add(x=w567, y=1) -> (x+y=w565:dbl[][])
      n357 = call <vilib>:"Create Occupancy Grid Map.vi"("occupancy grid"=w565) -> ("error out"=w564:errorcluster, "map reference out"=w560:refnum<data-value>)  [unwired: 9 in]
      n358 = Index Array(array=w555, index #1=0, index #2=1) -> (element #1=w545:dbl, element #2=w544:dbl)
      n359 = local read "target location"() -> (w552:dbl[])
      n360 = call <vilib>:"Get Cell Reference.vi"("error in (no error)"=w564, "y"=w545, "x"=w544, "map reference in"=w560) -> ("error out"=w563:errorcluster, "cell reference"=w561:refnum<data-value>, "map reference out"=w573:refnum<data-value>)  [unwired: 4 in, 1 out]
      n361 = Index Array(array=w552, index #1=0, index #2=1) -> (element #1=w549:dbl, element #2=w548:dbl)
      n362 = Decrement(x=w548) -> (x-1=w546:dbl)
      n363 = Decrement(x=w549) -> (x-1=w547:dbl)
      n364 = call <vilib>:"Get Cell Reference.vi"("error in (no error)"=w563, "y"=w547, "x"=w546, "map reference in"=w573) -> ("error out"=w562:errorcluster, "cell reference"=w559:refnum<data-value>, "map reference out"=w571:refnum<data-value>)  [unwired: 4 in, 1 out]
      n365 = call <vilib>:"A Star Plan.vi"("goal reference"=w559, "start reference"=w561, "map reference in"=w571) -> ("path references"=w572:refnum<data-value>[])  [unwired: 5 in, 3 out]
      n366 = call <vilib>:"Get Cells in Path.vi"("error in (no error)"=w562, "path references"=w572, "map reference in"=w571) -> ("error out"=w557:errorcluster, "y coordinates"=w570:i32[], "x coordinates"=w569:i32[], "map reference out"=w558:refnum<data-value>)  [unwired: 5 in]
      n367 = for {
        tunnel: w570 -> [w577] mode=indexing
        tunnel: w569 -> [w578] mode=indexing
        n368 = local read "Map"() -> (w574:u16[][])
        n369 = Replace Array Subset(array=w574, new element=2, index (row)=w578, index (col)=w577) -> (w575:u16[][])
        n370 = local write "Map"(w575) -> ()
      }
      n371 = call <vilib>:"Close Occupancy Grid Map.vi"("error in (no error)"=w557, "map reference in"=w558) -> ()  [unwired: 9 in, 1 out]
    }
    frame #12 {
      n372 = local read "robot location"() -> (w581:dbl[])
      n373 = local read "robot location"() -> (w582:dbl[])
      n374 = local read "Map"() -> (w583:u16[][])
      n375 = Index Array(array=w581, index=0) -> (element=w580:dbl)
      n376 = Index Array(array=w582, index=1) -> (element=w585:dbl)
      n377 = Replace Array Subset(array=w583, new element=5, index (row)=w585, index (col)=w580) -> (w584:u16[][])
      n378 = local write "Map"(w584) -> ()
    }
  }
